vi "Extract Waveform Parameters.vi"(8 "error in (no error)":errorcluster, 10 "RF Calibration Parameters In":T1[](array[typedef]), 11 "Measurement Interface":refnum<class "QPA Measurement.lvclass">) -> (0 "error out":errorcluster, 2 "RF Calibration Parameters Out":T1[](array[typedef]))   [LabVIEW 2016]
uses:
  Typedefs/RF Calibration Parameters.ctl
  Plugins/QPA Measurement.lvlibp/QPA Measurement.lvclass
  Plugins/QPA Measurement.lvlibp/Waveform Manager/Controls/RF Waveform.ctl
  Plugins/QPA Measurement.lvlibp/Waveform Manager/QPA MSMT Waveform Manager.lvclass
  niRFSTS Sequence Flow.lvclass
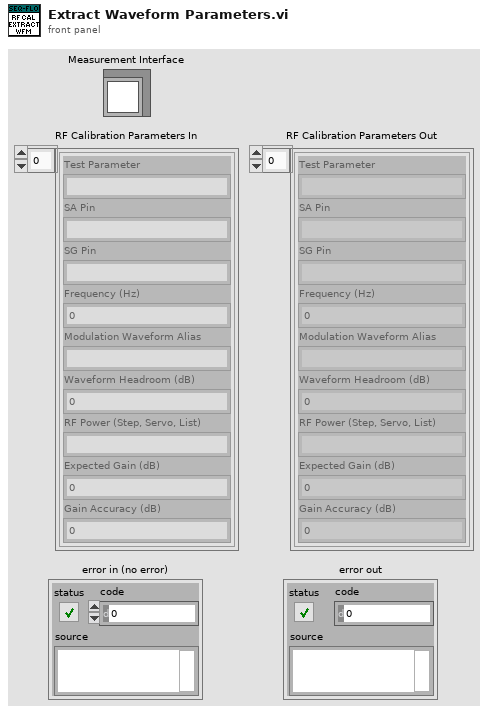
[diagram p1: front panel]
types:
  T1 = typedef "niRFSTS Sequence Flow.lvclass/RF Calibration Parameters.ctl" = cluster{"Test Parameter":string, "SA Pin":string, "SG Pin":string, "Frequency (Hz)":dbl, "Modulation Waveform Alias":string, "Waveform Headroom (dB)":dbl, "RF Power (Step, Servo, List)":string, "Expected Gain (dB)":dbl, "Gain Accuracy (dB)":dbl}
  T2 = typedef "QPA Measurement.lvlibp/QPA MSMT Waveform Manager.lvclass/RF Waveform.ctl" = cluster{"Name":string, "Path":path, "Headroom":dbl, "Burst Length":dbl}
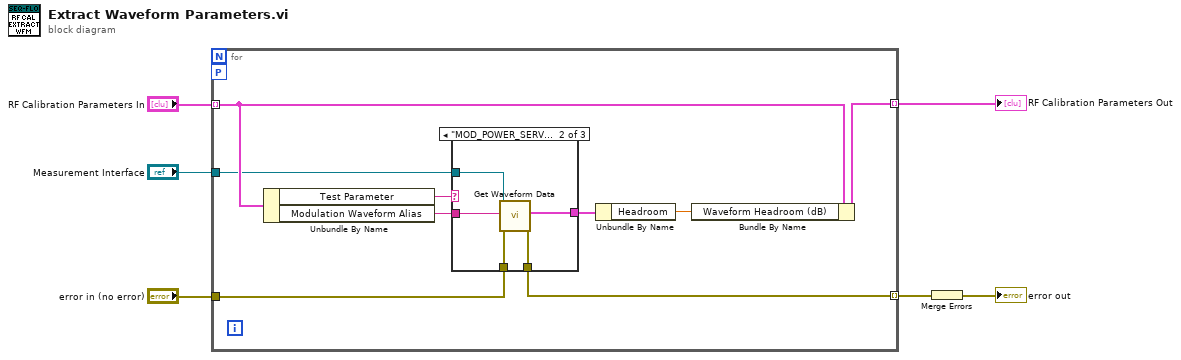
[diagram p0: block diagram]
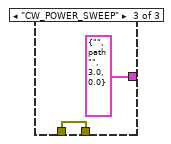
[diagram p3: hidden frame]
diagram:
  n1 = for {
    tunnel: [w14] -> w6 mode=indexing
    tunnel: "RF Calibration Parameters In" -> [w15] mode=indexing
    tunnel: "Measurement Interface" -> [w13]
    tunnel: "error in (no error)" -> [w12]
    tunnel: [w11] -> w2 mode=indexing
    workers-P: _ -> [_]
    n2 = Unbundle By Name(w15) -> ("Test Parameter"=w7:string, "Modulation Waveform Alias"=w10:string)
    n3 = case shown="\"MOD_POWER_SERVO\", \"MOD_POWER_SWEEP\"" w7 {
      tunnel: w13 -> [_ w21 _]
      tunnel: w12 -> [w16 w20 w22]
      tunnel: [w16 w19 w22] -> w11
      tunnel: w10 -> [_ w18 _]
      tunnel: [_ w17 T2 {"Name"="", "Path"=path "", "Headroom"=3.0, "Burst Length"=0.0} ("RF Waveform")] -> w8
      frame Default {
      }
      frame "MOD_POWER_SERVO", "MOD_POWER_SWEEP" {
        n4 = call "Get Waveform Data.vi"("error in (no error)"=w20, "Waveform to Retrieve"=w18, "QPA Measurement in"=w21) -> ("error out"=w19:errorcluster, "RF Waveform"=w17:T2)  [unwired: 6 in, 1 out]
      }
      frame "CW_POWER_SWEEP" {
      }
    }
    n5 = Unbundle By Name(w8) -> ("Headroom"=w9:dbl)
    n6 = Bundle By Name(cluster=w15, "Waveform Headroom (dB)"=w9) -> (w14:T1)
  }
  "RF Calibration Parameters Out" <- w6
  n7 = Merge Errors(w2) -> (→"error out":errorcluster)
